vi "Stop.vi"(8 "error in":errorcluster, 11 "HL Timer in":refnum<class "Loop Timer.lvclass">) -> (0 "error out":errorcluster, 3 "HL Timer out":refnum<class "Loop Timer.lvclass">)   [LabVIEW 2022 SP3, in "hse-misc.lvlib" / "Loop Timer.lvclass"]
doc: "Stop the timed loop by setting the event timeout to \"-1\".\n\n____\nHAMPEL SOFTWARE ENGINEERING v3.8.0 (2023-12-18 14:41)"
uses:
  Loop Timer.lvclass
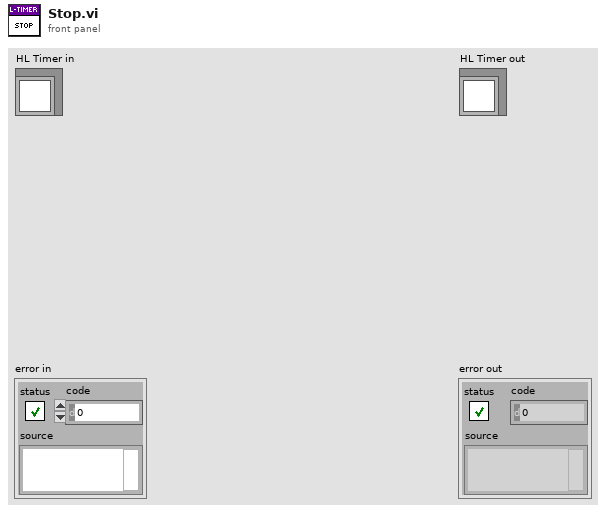
[diagram p1: front panel]
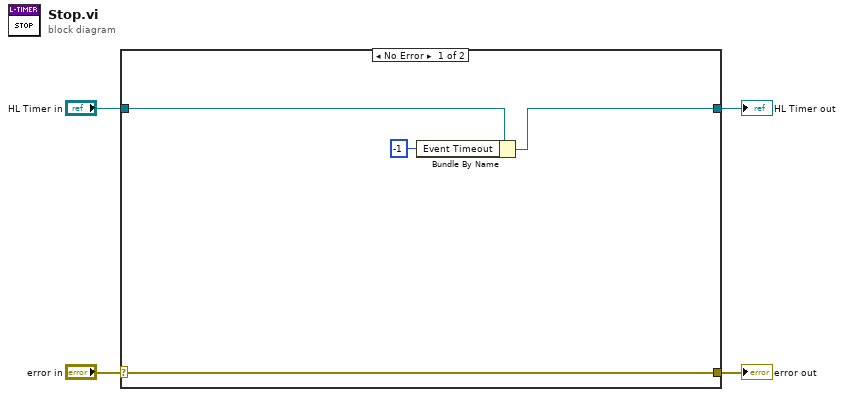
[diagram p0: block diagram]
diagram:
  n1 = case shown="No Error" "error in" {
    selector: "error in" -> [w7 w10]
    tunnel: [w7 w10] -> w3
    tunnel: [w6 w9] -> w1
    tunnel: "HL Timer in" -> [w8 w9]
    frame No Error {
      n2 = Bundle By Name(cluster=w8, "Event Timeout"=-1) -> (w6:refnum<class "Loop Timer.lvclass">)
    }
    frame Error {
    }
  }
  "error out" <- w3
  "HL Timer out" <- w1
